vi "9_sub_MoveY_N.vi"(6 "Dir":string, 8 "T_y":i32, 9 "T_x":i32, 10 "H_y":i32, 11 "H_x":i32) -> (2 "T_y 2":i32, 3 "T_x 2":i32, 5 "H_y 2":i32, 7 "H_x 2":i32)   [LabVIEW 2021, in "2022.lvlib"]
uses:
  2022.lvlib
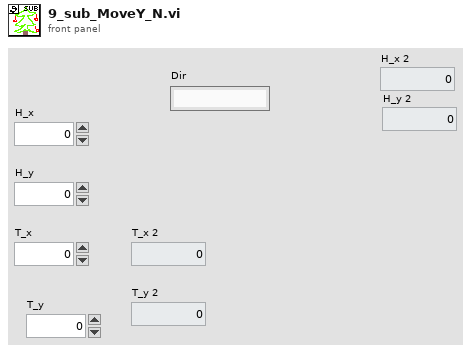
[diagram p1: front panel]
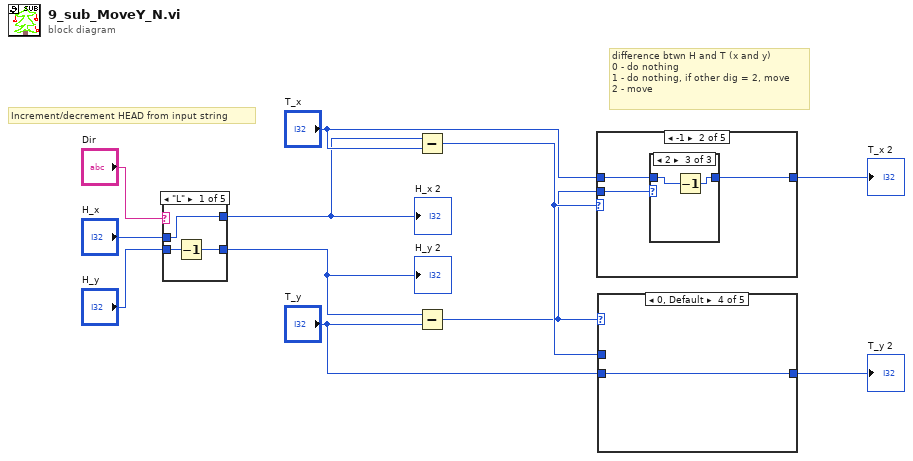
[diagram p0: block diagram]
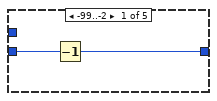
[diagram p2: hidden frame]
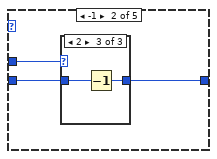
[diagram p3: hidden frame]
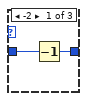
[diagram p4: hidden frame]
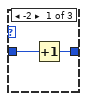
[diagram p7: hidden frame]
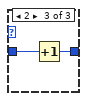
[diagram p8: hidden frame]
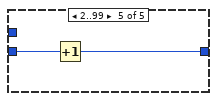
[diagram p9: hidden frame]
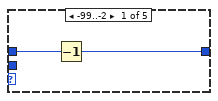
[diagram p10: hidden frame]
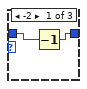
[diagram p11: hidden frame]
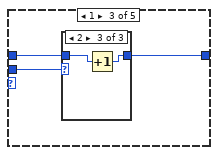
[diagram p13: hidden frame]
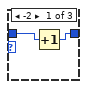
[diagram p14: hidden frame]
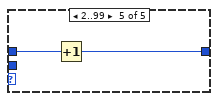
[diagram p17: hidden frame]
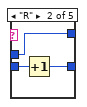
[diagram p18: hidden frame]
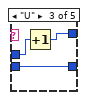
[diagram p19: hidden frame]
diagram:
  # "difference btwn H and T (x and y)\n0 - do nothing\n1 - do nothing, if other dig = 2, move\n2 - move"
  # "Increment/decrement HEAD from input string"
  n1 = case shown="\"L\"" "Dir" {
    tunnel: "H_y" -> [w13 w17 w18 w21 w25]
    tunnel: [w12 w16 w18 w21 w25] -> w2
    tunnel: "H_x" -> [w14 w15 w20 w22 w24]
    tunnel: [w14 w15 w19 w22 w23] -> w3
    frame "L" {
      n2 = Decrement(x=w13) -> (x-1=w12:i32)
    }
    frame "R" {
      n3 = Increment(x=w17) -> (x+1=w16:i32)
    }
    frame "U" {
      n4 = Increment(x=w20) -> (x+1=w19:i32)
    }
    frame Default {
    }
    frame "D" {
      n5 = Decrement(x=w24) -> (x-1=w23:i32)
    }
  }
  "H_x 2" <- w3
  "H_y 2" <- w2
  n6 = Subtract(x=w3, y="T_x") -> (x-y=w7:i32)
  n7 = Subtract(x=w2, y="T_y") -> (x-y=w6:i32)
  n8 = case shown="-1" w7 {
    tunnel: "T_x" -> [w27 w29 w37 w44 w46]
    tunnel: [w26 w28 w36 w44 w45] -> w10
    tunnel: w6 -> [_ w30 w38 _ _]
    frame -99..-2 {
      n9 = Decrement(x=w27) -> (x-1=w26:i32)
    }
    frame -1 {
      n10 = case shown="2" w30 {
        tunnel: w29 -> [w32 w33 w35]
        tunnel: [w31 w33 w34] -> w28
        frame -2 {
          n11 = Decrement(x=w32) -> (x-1=w31:i32)
        }
        frame 0, Default {
        }
        frame 2 {
          n12 = Decrement(x=w35) -> (x-1=w34:i32)
        }
      }
    }
    frame 1 {
      n13 = case shown="2" w38 {
        tunnel: w37 -> [w40 w41 w43]
        tunnel: [w39 w41 w42] -> w36
        frame -2 {
          n14 = Increment(x=w40) -> (x+1=w39:i32)
        }
        frame 0, Default {
        }
        frame 2 {
          n15 = Increment(x=w43) -> (x+1=w42:i32)
        }
      }
    }
    frame 0, Default {
    }
    frame 2..99 {
      n16 = Increment(x=w46) -> (x+1=w45:i32)
    }
  }
  "T_x 2" <- w10
  n17 = case shown="0, Default" w6 {
    tunnel: "T_y" -> [w48 w50 w58 w65 w67]
    tunnel: [w47 w49 w57 w65 w66] -> w8
    tunnel: w7 -> [_ w51 w59 _ _]
    frame -99..-2 {
      n18 = Decrement(x=w48) -> (x-1=w47:i32)
    }
    frame -1 {
      n19 = case shown="2" w51 {
        tunnel: w50 -> [w53 w54 w56]
        tunnel: [w52 w54 w55] -> w49
        frame -2 {
          n20 = Decrement(x=w53) -> (x-1=w52:i32)
        }
        frame 0, Default {
        }
        frame 2 {
          n21 = Decrement(x=w56) -> (x-1=w55:i32)
        }
      }
    }
    frame 1 {
      n22 = case shown="0, Default" w59 {
        tunnel: w58 -> [w61 w62 w64]
        tunnel: [w60 w62 w63] -> w57
        frame -2 {
          n23 = Increment(x=w61) -> (x+1=w60:i32)
        }
        frame 0, Default {
        }
        frame 2 {
          n24 = Increment(x=w64) -> (x+1=w63:i32)
        }
      }
    }
    frame 0, Default {
    }
    frame 2..99 {
      n25 = Increment(x=w67) -> (x+1=w66:i32)
    }
  }
  "T_y 2" <- w8
